vi "TestPVCam_basic.vi"() -> ()   [LabVIEW 2022 SP3, in "Photometrics Camera.lvlib"]
uses:
  Photometrics Camera.lvlib
  cbc77bd3-37df-4bf8-83b9-1019cab143c6.vi
  C:/FlashGordon/Development/dll/PVCamNET.dll
  dll/PVCamNET.dll
panel:
  out "error out":errorcluster
  in  "Exposure time":u32=20
  out "SN":string
  out "CapturedFrames":u32
  out "output array":u16[][](array[numeric])
  in  "STOP":bool
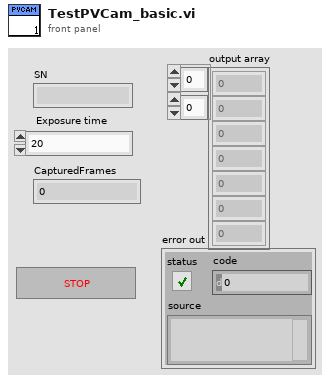
[diagram p1: front panel]
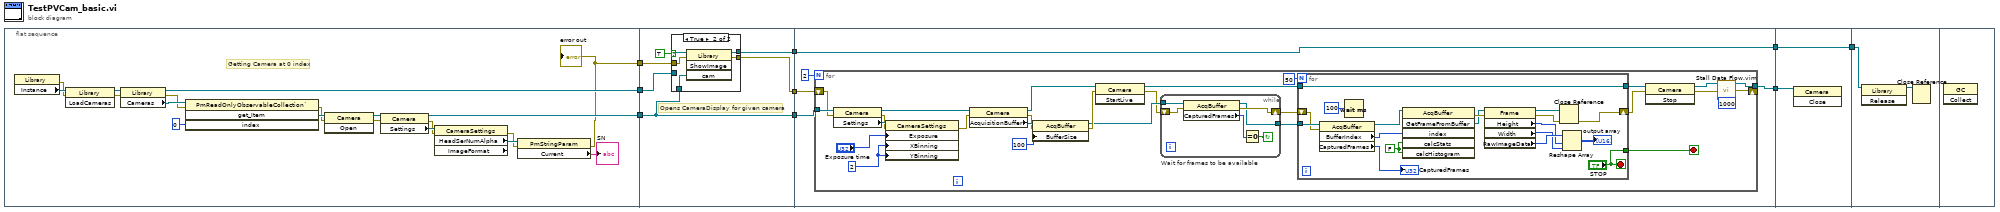
[diagram p0: block diagram]
diagram:
  n1 = flat-sequence {
    tunnel: [w25] -> w9
    tunnel: [w21] -> w8
    tunnel: [w10] -> w1
    tunnel: w9 -> [w34]
    tunnel: [w33] -> w4
    tunnel: w8 -> [w31]
    tunnel: [w31] -> w3
    tunnel: [w30] -> w2
    tunnel: w1 -> [w29]
    tunnel: [w46] -> w7
    tunnel: [w44] -> w5
    tunnel: w4 -> [w46]
    tunnel: w3 -> [w43]
    tunnel: w2 -> [w42]
    tunnel: w7 -> [w98]
    tunnel: [w98] -> w6
    tunnel: w5 -> [w97]
    tunnel: w6 -> [w100]
    frame #0 {
      # "Getting Camera at 0 index"
      n2 = property class="Library"() -> (error out=w17:errorcluster, "Instance"=w24:refnum<k24>)  [unwired: 2 in, 1 out]
      n3 = invoke class="Library" method="LoadCameras"(reference=w24, error in=w17) -> (reference out=w23:refnum<k24>, error out=w16:errorcluster)  [unwired: 1 in, 1 out]
      n4 = property class="Library"(reference=w23, error in=w16) -> (reference out=w25:refnum<k24>, error out=w15:errorcluster, "Cameras"=w28:refnum<k24>)
      n5 = invoke class="PmReadOnlyObservableCollection`" method="get_Item"(reference=w28, error in=w15, "index"=0) -> (error out=w14:errorcluster, "get_Item"=w26:refnum<k24>)  [unwired: 1 in, 2 out]
      n6 = invoke class="Camera" method="Open"(reference=w26, error in=w14) -> (reference out=w22:refnum<k24>, error out=w13:errorcluster)  [unwired: 1 in, 1 out]
      n7 = property class="Camera"(reference=w22, error in=w13) -> (reference out=w21:refnum<k24>, error out=w12:errorcluster, "Settings"=w20:refnum<k24>)
      n8 = property class="CameraSettings" props=["HeadSerNumAlpha", "ImageFormat"](reference=w20, error in=w12) -> (error out=w11:errorcluster, "HeadSerNumAlpha"=w19:refnum<k24>)  [unwired: 2 out]
      n9 = property class="PmStringParam"(reference=w19, error in=w11) -> (error out=w10:errorcluster, "Current"=→"SN":string)  [unwired: 1 out]
      "error out" <- w10
    }
    frame #1 {
      # "Opens CameraDisplay for given camera"
      n10 = case shown="True" TRUE {
        tunnel: w34 -> [w36 w41]
        tunnel: [w36 w40] -> w33
        tunnel: w31 -> [_ w39]
        tunnel: [w35 w38] -> w30
        tunnel: w29 -> [w35 w37]
        frame False {
        }
        frame True {
          n11 = invoke class="Library" method="ShowImage"(reference=w41, error in=w37, "cam"=w39) -> (reference out=w40:refnum<k24>, error out=w38:errorcluster)  [unwired: 1 in, 2 out]
        }
      }
    }
    frame #2 {
      n12 = for {
        N: 2 -> [_]
        tunnel: [w49] -> w44
        tunnel: w43 -> [w69]
        shift-right: [w50] -> _
        shift-left: w42 -> [w61]
        stop <- w71 stop-if-true
        w47 = u16 2 ("XBinning")
        n13 = property class="Camera"(reference=w69, error in=w61) -> (reference out=w60:refnum<k24>, error out=w64:errorcluster, "Settings"=w65:refnum<k24>)
        n14 = property class="CameraSettings"(reference=w65, error in=w64, "Exposure"="Exposure time", "XBinning"=w47, "YBinning"=w47) -> (error out=w59:errorcluster)  [unwired: 1 out]
        n15 = property class="Camera"(reference=w60, error in=w59) -> (reference out=w58:refnum<k24>, error out=w63:errorcluster, "AcquisitionBuffer"=w67:refnum<k24>)
        n16 = property class="AcqBuffer"(reference=w67, error in=w63, "BufferSize"=u32 100) -> (reference out=w55:refnum<k24>, error out=w56:errorcluster)
        n17 = invoke class="Camera" method="StartLive"(reference=w58, error in=w56) -> (reference out=w57:refnum<k24>, error out=w53:errorcluster)  [unwired: 1 in, 1 out]
        n18 = while "Wait for frames to be available" {
          shift-right: [w77] -> w54
          shift-left: w53 -> [w78]
          tunnel: [w74] -> w52
          tunnel: w55 -> [w73]
          stop <- w75 continue-if-true
          n19 = property class="AcqBuffer"(reference=w73, error in=w78) -> (reference out=w74:refnum<k24>, error out=w77:errorcluster, "CapturedFrames"=w76:u32)
          n20 = Equal To 0?(x=w76) -> (x = 0?=w75:bool)
        }
        n21 = for {
          N: 50 -> [_]
          tunnel: w52 -> [w90]
          tunnel: ["STOP"] -> w71
          tunnel: [w88] -> w70
          tunnel: w57 -> [w88]
          shift-right: [w85] -> w62
          shift-left: w54 -> [w87]
          stop <- "STOP" stop-if-true
          w81 = FALSE ("calcStats")
          n22 = property class="AcqBuffer"(reference=w90, error in=w87) -> (reference out=w83:refnum<k24>, "BufferIndex"=w79:u32, "CapturedFrames"=→"CapturedFrames":u32)  [unwired: 1 out]
          n23 = Wait (ms)(milliseconds to wait=u32 100) -> ()  [unwired: 1 out]
          n24 = invoke class="AcqBuffer" method="GetFrameFromBuffer"(reference=w83, "index"=w79, "calcStats"=w81, "calcHistogram"=w81) -> (error out=w84:errorcluster, "GetFrameFromBuffer"=w82:refnum<k24>)  [unwired: 2 in, 4 out]
          n25 = property class="Frame"(reference=w82, error in=w84) -> (reference out=w92:refnum<k24>, error out=w86:errorcluster, "Height"=w93:u32, "Width"=w94:u32, "RawImageData"=w95:u16[])
          n26 = Close Reference(reference=w92, error in (no error)=w86) -> (error out=w85:errorcluster)
          n27 = Reshape Array(w95, w93, w94) -> (→"output array":u16[][])
        }
        n28 = invoke class="Camera" method="Stop"(reference=w70, error in=w62) -> (reference out=w49:refnum<k24>, error out=w51:errorcluster)  [unwired: 1 in, 1 out]
        n29 = call "Stall Data Flow.vim"("value in"=w51, "milliseconds to wait"=u32 1000) -> ("value out"=w50:errorcluster)  [unwired: 1 out]
      }
    }
    frame #3 {
      n30 = invoke class="Camera" method="Close"(reference=w97) -> ()  [unwired: 2 in, 3 out]
    }
    frame #4 {
      n31 = invoke class="Library" method="Release"(reference=w100) -> (reference out=w99:refnum<k24>)  [unwired: 2 in, 2 out]
      n32 = Close Reference(reference=w99) -> ()  [unwired: 1 in, 1 out]
    }
    frame #5 {
      n33 = invoke class="GC" method="Collect"() -> ()  [unwired: 3 in, 3 out]
    }
  }
